vi "Vessel Operation.vi"() -> ()   [LabVIEW 2017, in "Saturation.lvclass"]
uses:
  Saturation.lvclass
  Type Defs/Tank.ctl
  Type Defs/Saturation State.ctl
  Process Settings/Process Settings.lvclass
  Process Settings/Type Defs/Item.ctl
  Type Defs/Valve State.ctl
  Process Settings/Type Defs/Units.ctl
panel:
  out "Elapsed Time":dbl(slide) scale=0.0..60.0
  in  "Stop":bool
  in  "Start":bool
  out "Temperature (bottom)":dbl
  out "Temperature (middle)":dbl
  out "Temperature (top)":dbl
  in  "Pressure Sensor Enabled":bool
  in  "Temperature (bottom) Enabled":bool
  in  "Temperature (middle) Enabled":bool
  in  "Temperature (top) Enabled":bool
  out "Tank pressure":T1 scale=0.0..100.0
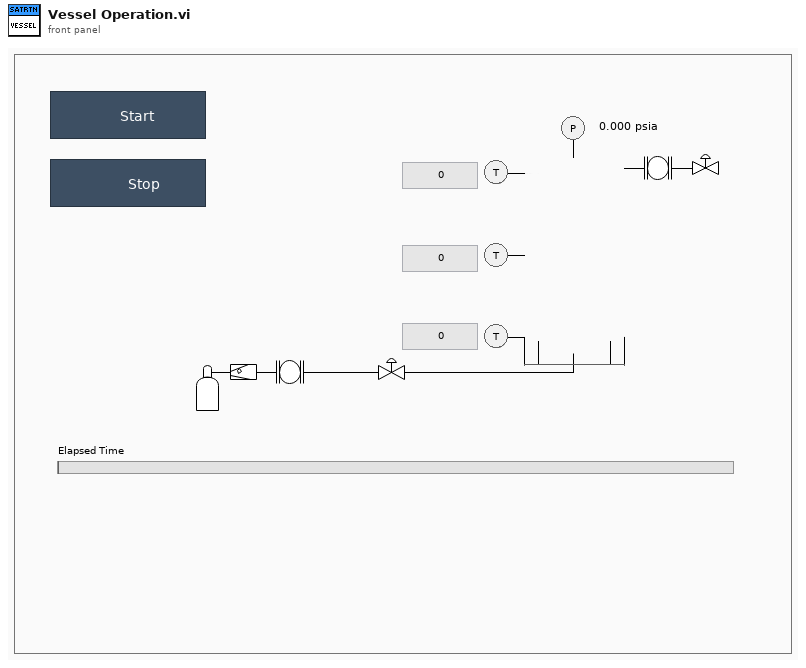
[diagram p1: front panel]
types:
  T1 = typedef "Saturation.lvclass/Tank.ctl" = dbl
  T2 = typedef "Saturation.lvclass/Saturation State.ctl" = enum16{"Init", "Update", "Go", "Control Valve", "Wait for Pressure", "Wait and Monitor", "Stop", "Idle", "Error", "Shutdown"}
  T3 = enum32{"Bad", "Idle", "Run top level", "Running"}
  T4 = typedef "Saturation.lvclass/Valve State.ctl" = enum16{"Fill", "Saturate", "Exhaust"}
  T5 = typedef "Process Settings.lvclass/Item.ctl" = enum16{"", "sheet temperature setpoint", "sheet heating time", "temp element setpoint", "chamber pressure setpoint", "saturation time", "chamber pressure valve setpoint"}
  T6 = typedef "Process Settings.lvclass/Units.ctl" = enum16{"°F", "°C", "Seconds", "Minutes", "PSIA", "V"}
  T7 = typedef "Saturation.lvclass/Saturation Temps.ctl" = cluster{"Tank Top Temp":dbl, "Tank Middle Temp":dbl, "Tank Bottom Temp":dbl}
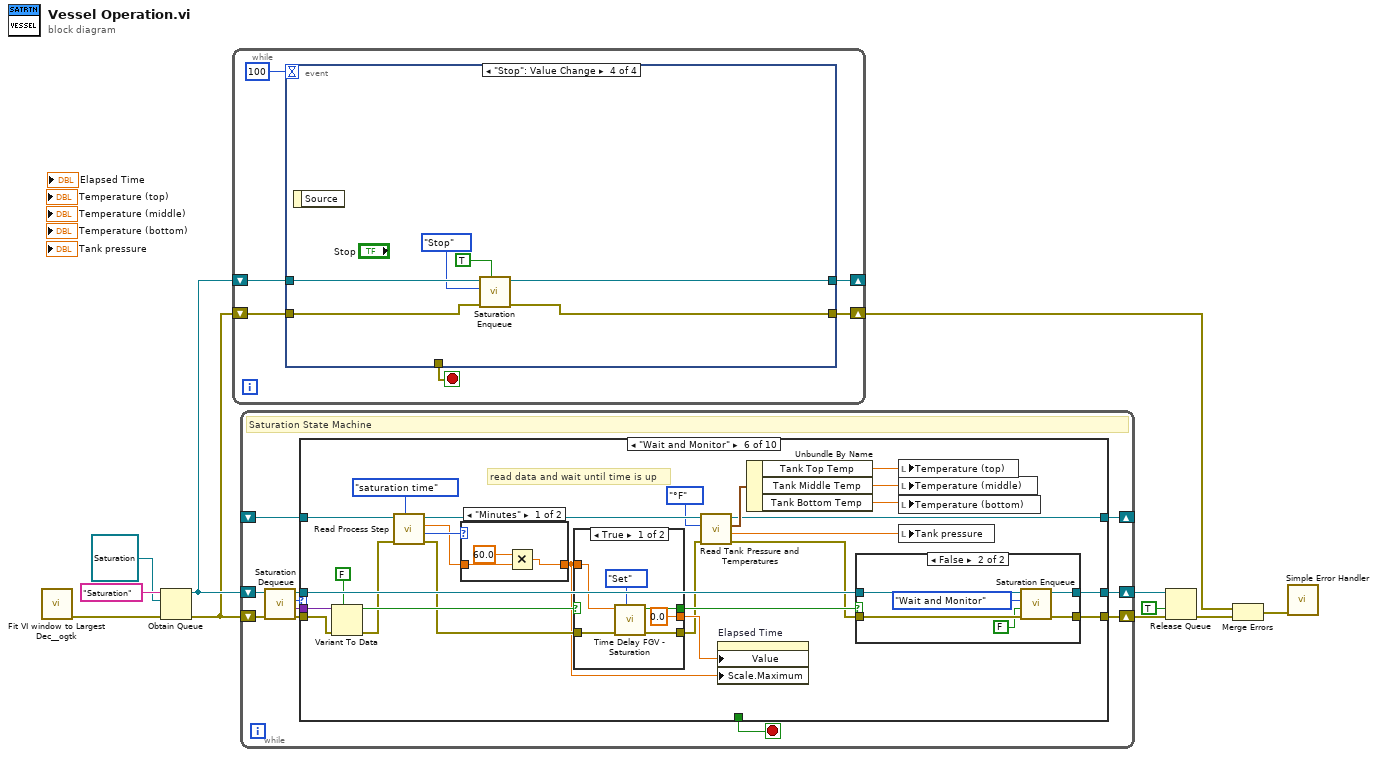
[diagram p0: block diagram]
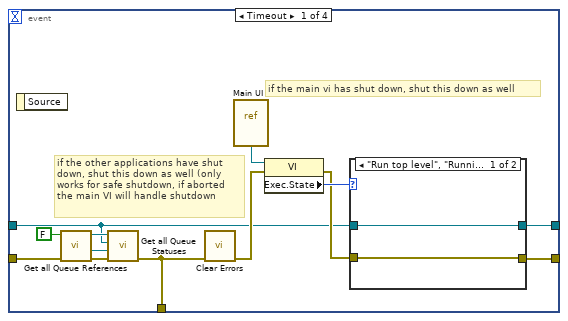
[diagram p2: hidden frame]
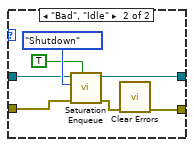
[diagram p3: hidden frame]
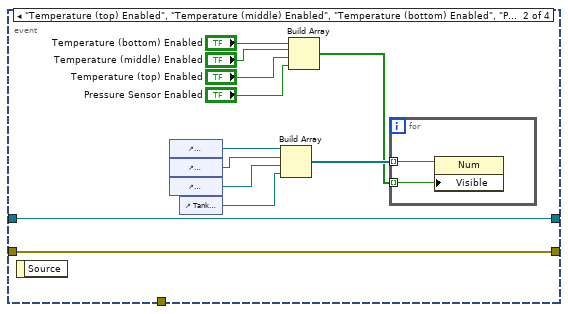
[diagram p4: hidden frame]
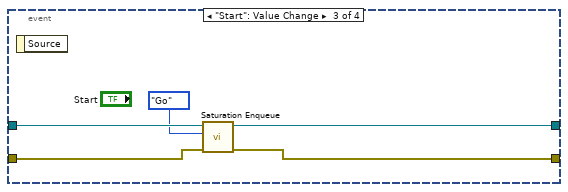
[diagram p5: hidden frame]
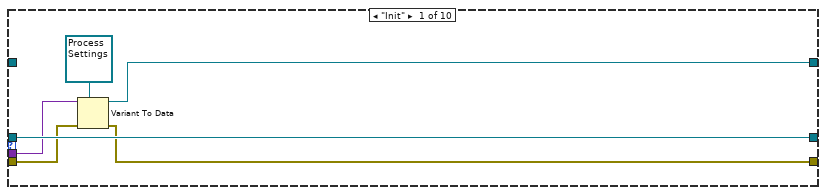
[diagram p6: hidden frame]
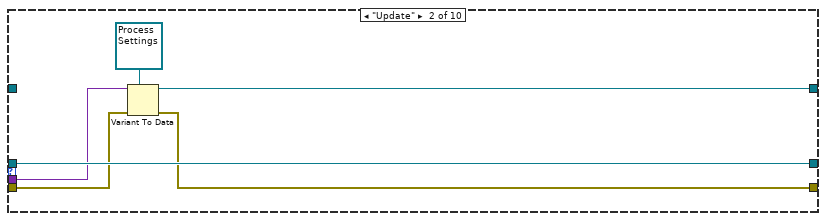
[diagram p7: hidden frame]
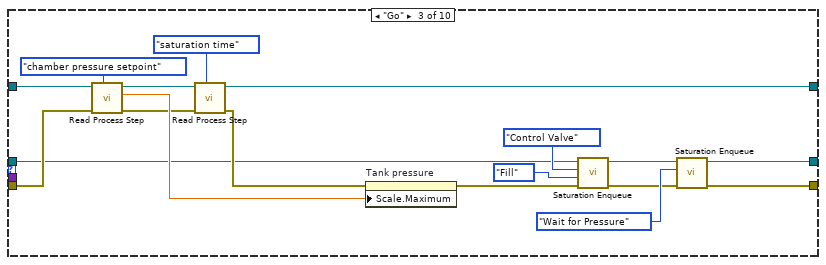
[diagram p8: hidden frame]
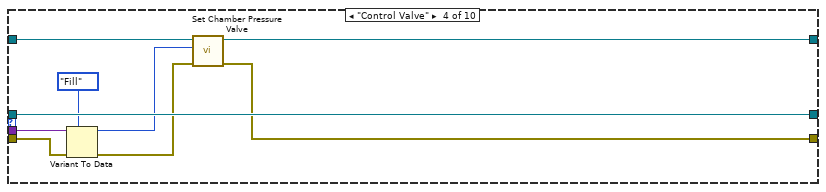
[diagram p9: hidden frame]
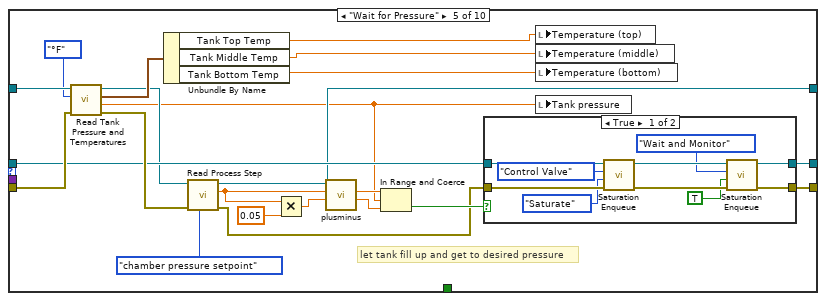
[diagram p10: hidden frame]
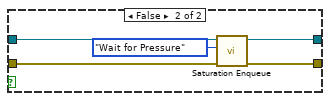
[diagram p11: hidden frame]
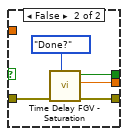
[diagram p13: hidden frame]
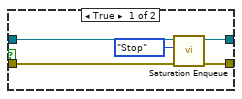
[diagram p14: hidden frame]
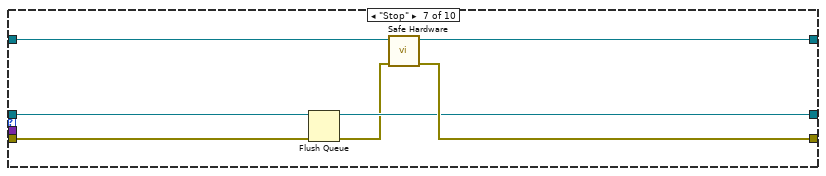
[diagram p15: hidden frame]
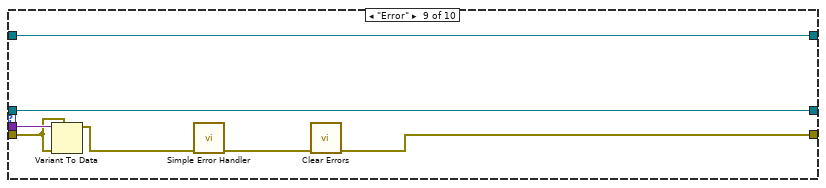
[diagram p17: hidden frame]
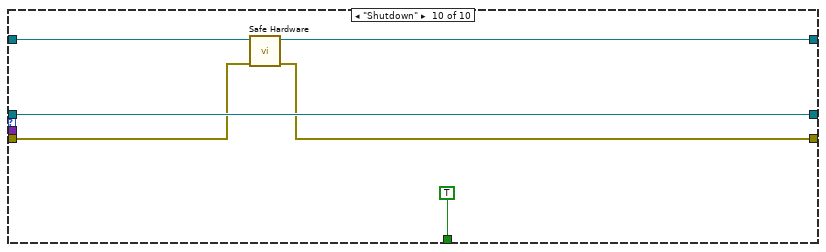
[diagram p18: hidden frame]
diagram:
  n1 = call <userlib>:"Fit VI window to Largest Dec__ogtk.vi"() -> ("error out"=w8:errorcluster)  [unwired: 6 in, 1 out]
  n2 = Obtain Queue(name (unnamed)="Saturation", element data type=refnum<class "Saturation.lvclass"> refnum ("Expansion.lvclass"), error in (no error)=w8) -> (queue out=w5:refnum<queue>, error out=w1:errorcluster)  [unwired: 2 in, 1 out]
  n3 = while {
    shift-right: [w14] -> w3
    shift-left: w1 -> [w16]
    shift-right: [w13] -> _
    shift-left: w5 -> [w17]
    stop <- w15 stop-if-true
    n4 = event shown="[3] \"Stop\": Value Change" {
      selector: _ -> [_ _ _ _]
      dyn-events: _ -> [_ _ _ _]
      timeout: 100 -> [_ _ _ _]
      tunnel: w17 -> [w19 w50 w58 w64]
      tunnel: w16 -> [w26 w51 w56 w62]
      tunnel: [w18 _ _ _] -> w15
      tunnel: [w20 w51 w55 w61] -> w14
      tunnel: [w21 w50 w57 w63] -> w13
      event Timeout {
        # "if the other applications have shut down, shut this down as well (only works for safe shutdown, if aborted the main VI will handle shutdown"
        # "if the main vi has shut down, shut this down as well"
        n5 = event-data() -> ()  [unwired: 1 in, 1 out]
        n6 = call "Get all Queue References.vi"("error in (no error)"=w26, "create if not found? (F)"=FALSE ("create if not found? (T)")) -> ("error out"=w29:errorcluster, "Recipes Queue"=w30:refnum<queue>, "Expansion Queue"=w27:refnum<queue>)  [unwired: 6 in, 1 out]
        n7 = call "Get all Queue Statuses.vi"("error in (no error)"=w29, "Recipes Queue"=w30, "Saturation Queue"=w19, "Expansion Queue"=w27) -> ("error out"=w18:errorcluster)  [unwired: 7 in]
        n8 = call <vilib>:"Clear Errors.vi"("error in (no error)"=w18) -> ("error out"=w23:errorcluster)  [unwired: 5 in, 1 out]
        n9 = vi-ref "Main UI.vi"() -> (w25:refnum<vi>)
        n10 = property class="VI"(reference=w25, error in=w23) -> (error out=w22:errorcluster, "Exec.State"=w24:T3)  [unwired: 1 out]
        n11 = case shown="\"Run top level\", \"Running\"" w24 {
          tunnel: w19 -> [w32 w35]
          tunnel: [w32 w39] -> w21
          tunnel: [w31 w33] -> w20
          tunnel: w22 -> [w31 w37]
          frame "Run top level", "Running" {
          }
          frame "Bad", "Idle" {
            n12 = call "Saturation Enqueue.vi"("Opposite End?"=TRUE, "error in (no error)"=w37, "State"=Saturation_State."Shutdown", "Queue in"=w35) -> ("error out"=w38:errorcluster, "Queue out"=w39:refnum<queue>)  [unwired: 6 in]
            n13 = call <vilib>:"Clear Errors.vi"("error in (no error)"=w38) -> ("error out"=w33:errorcluster)  [unwired: 5 in, 1 out]
          }
        }
      }
      event "Temperature (top) Enabled", "Temperature (middle) Enabled", "Temperature (bottom) Enabled", "Pressure Sensor Enabled": Value Change {
        n14 = event-data() -> ()  [unwired: 1 in, 1 out]
        n15 = control-ref of="Temperature (bottom)"() -> (w49:refnum<vi>)
        n16 = control-ref of="Temperature (middle)"() -> (w48:refnum<vi>)
        n17 = control-ref of="Temperature (top)"() -> (w47:refnum<vi>)
        n18 = control-ref of="Tank pressure"() -> (w46:refnum<vi>)
        n19 = Build Array(w49, w48, w47, w46) -> (w41:refnum<vi>[])
        n20 = Build Array("Temperature (bottom) Enabled", "Temperature (middle) Enabled", "Temperature (top) Enabled", "Pressure Sensor Enabled") -> (w40:bool[])
        n21 = for {
          tunnel: w41 -> [w53] mode=indexing
          tunnel: w40 -> [w52] mode=indexing
          n22 = property class="Num"(reference=w53, "Visible"=w52) -> ()  [unwired: 1 in, 2 out]
        }
      }
      event "Start": Value Change {
        n23 = event-data() -> ()  [unwired: 1 in, 1 out]
        n24 = call "Saturation Enqueue.vi"("error in (no error)"=w56, "State"=Saturation_State."Go", "Queue in"=w58) -> ("error out"=w55:errorcluster, "Queue out"=w57:refnum<queue>)  [unwired: 7 in]
      }
      event "Stop": Value Change {
        n25 = event-data() -> ()  [unwired: 1 in, 1 out]
        n26 = call "Saturation Enqueue.vi"("Opposite End?"=TRUE, "error in (no error)"=w62, "State"=Saturation_State."Stop", "Queue in"=w64) -> ("error out"=w61:errorcluster, "Queue out"=w63:refnum<queue>)  [unwired: 6 in]
      }
    }
  }
  n27 = while {
    shift-right: [w71] -> w10
    shift-left: w1 -> [w74]
    shift-right: [w69] -> w11
    shift-left: w5 -> [w75]
    shift-right: [w66] -> _
    shift-left: _ -> [w65]
    stop <- w70 stop-if-true
    # "Saturation State Machine"
    n28 = call "Saturation Dequeue.vi"("error in (no error)"=w74, "Queue in"=w75) -> ("error out"=w72:errorcluster, "Data"=w67:variant, "State"=w68:T2, "Queue out"=w73:refnum<queue>)  [unwired: 6 in]
    n29 = case shown="\"Wait and Monitor\"" w68 {
      tunnel: w73 -> [w81 w87 w95 w114 w120 w177 w210 w212 w220 w226]
      tunnel: w72 -> [w77 w82 w105 w111 w135 w173 w205 w213 w216 w222]
      tunnel: [w76 w84 w90 w107 w125 w175 w207 w213 w219 w221] -> w71
      tunnel: [_ _ _ _ _ _ _ _ _ TRUE] -> w70
      tunnel: [w81 w87 w92 w114 w126 w176 w206 w212 w220 w226] -> w69
      tunnel: w67 -> [w79 w85 _ w113 _ w174 _ _ w218 _]
      tunnel: [w78 w83 w98 w108 w117 w157 w208 w211 w215 w223] -> w66
      tunnel: w65 -> [_ _ w99 w109 w134 w168 w209 w211 w215 w224]
      frame "Init" {
        n30 = Variant To Data(error in=w77, type=refnum<class "Process Settings.lvclass"> refnum ("Process Settings.lvclass"), Variant=w79) -> (data=w78:refnum<class "Process Settings.lvclass">, error out=w76:errorcluster)
      }
      frame "Update" {
        n31 = Variant To Data(error in=w82, type=refnum<class "Process Settings.lvclass"> refnum ("Process Settings.lvclass"), Variant=w85) -> (data=w83:refnum<class "Process Settings.lvclass">, error out=w84:errorcluster)
      }
      frame "Go" {
        n32 = call "Read Process Step.vi"("Item"=Item."chamber pressure setpoint", "error in (no error)"=w105, "Process Settings in"=w99) -> ("error out"=w97:errorcluster, "Value"=w103:dbl, "Process Settings out"=w101:refnum<class "Process Settings.lvclass">)  [unwired: 5 in, 1 out]
        n33 = call "Read Process Step.vi"("Item"=Item."saturation time", "error in (no error)"=w97, "Process Settings in"=w101) -> ("error out"=w96:errorcluster, "Process Settings out"=w98:refnum<class "Process Settings.lvclass">)  [unwired: 5 in, 2 out]
        n34 = property on="Tank pressure" class="Slide (strict)"(error in=w96, "Scale.Maximum"=w103) -> (error out=w94:errorcluster)  [unwired: 1 in, 1 out]
        n35 = call "Saturation Enqueue.vi"("error in (no error)"=w94, "Data"=Valve_State."Fill" ("Open/Closed"), "State"=Saturation_State."Control Valve", "Queue in"=w95) -> ("error out"=w89:errorcluster, "Queue out"=w93:refnum<queue>)  [unwired: 6 in]
        n36 = call "Saturation Enqueue.vi"("error in (no error)"=w89, "State"=Saturation_State."Wait for Pressure", "Queue in"=w93) -> ("error out"=w90:errorcluster, "Queue out"=w92:refnum<queue>)  [unwired: 7 in]
      }
      frame "Control Valve" {
        n37 = Variant To Data(error in=w111, type=Valve_State."Fill" ("Open/Closed"), Variant=w113) -> (data=w110:T4, error out=w106:errorcluster)
        n38 = call "Set Chamber Pressure Valve.vi"("error in (no error)"=w106, "State"=w110, "Process Settings in"=w109) -> ("error out"=w107:errorcluster, "Process Settings out"=w108:refnum<class "Process Settings.lvclass">)  [unwired: 7 in]
      }
      frame "Wait for Pressure" {
        # "let tank fill up and get to desired pressure"
        n39 = call "Read Tank Pressure and Temperatures.vi"("error in (no error)"=w135, "Temp Units"=Units."°F", "Process Settings in"=w134) -> ("error out"=w121:errorcluster, "Tank Pressure"=w115:dbl, "Tank Temperature Cluster"=w136:T7, "Process Settings out"=w118:refnum<class "Process Settings.lvclass">)  [unwired: 5 in]
        n40 = Unbundle By Name(w136) -> ("Tank Top Temp"=w122:dbl, "Tank Middle Temp"=w123:dbl, "Tank Bottom Temp"=w124:dbl)
        n41 = call "Read Process Step.vi"("Item"=Item."chamber pressure setpoint", "error in (no error)"=w121, "Process Settings in"=w118) -> ("error out"=w119:errorcluster, "Value"=w130:dbl, "Process Settings out"=w117:refnum<class "Process Settings.lvclass">)  [unwired: 5 in, 1 out]
        n42 = Multiply(x=w130, y=0.05) -> (x*y=w131:dbl)
        n43 = call "plusminus.vi"("y"=w131, "x"=w130) -> ("x - y"=w128:dbl, "x + y"=w129:dbl)  [unwired: 4 in]
        n44 = In Range and Coerce(upper limit=w129, x=w115, lower limit=w128) -> (In Range?=w127:bool)  [unwired: 1 out]
        n45 = case shown="True" w127 {
          tunnel: w120 -> [w146 w151]
          tunnel: [w141 w150] -> w126
          tunnel: w119 -> [w145 w149]
          tunnel: [w140 w148] -> w125
          frame True {
            n46 = call "Saturation Enqueue.vi"("error in (no error)"=w145, "Data"=Valve_State."Saturate" ("Open/Closed"), "State"=Saturation_State."Control Valve", "Queue in"=w146) -> ("error out"=w139:errorcluster, "Queue out"=w142:refnum<queue>)  [unwired: 6 in]
            n47 = call "Saturation Enqueue.vi"("error in (no error)"=w139, "Data"=TRUE, "State"=Saturation_State."Wait and Monitor", "Queue in"=w142) -> ("error out"=w140:errorcluster, "Queue out"=w141:refnum<queue>)  [unwired: 6 in]
          }
          frame False {
            n48 = call "Saturation Enqueue.vi"("error in (no error)"=w149, "State"=Saturation_State."Wait for Pressure", "Queue in"=w151) -> ("error out"=w148:errorcluster, "Queue out"=w150:refnum<queue>)  [unwired: 7 in]
          }
        }
        n49 = local write "Temperature (top)"(w122) -> ()
        n50 = local write "Temperature (middle)"(w123) -> ()
        n51 = local write "Temperature (bottom)"(w124) -> ()
        n52 = local write "Tank pressure"(w115) -> ()
      }
      frame "Wait and Monitor" {
        # "read data and wait until time is up"
        n53 = Variant To Data(error in=w173, type=FALSE, Variant=w174) -> (data=w170:bool, error out=w167:errorcluster)
        n54 = call "Read Process Step.vi"("Item"=Item."saturation time", "error in (no error)"=w167, "Process Settings in"=w168) -> ("error out"=w166:errorcluster, "Units"=w160:T6, "Value"=w159:dbl, "Process Settings out"=w158:refnum<class "Process Settings.lvclass">)  [unwired: 5 in]
        n55 = case shown="\"Minutes\"" w160 {
          tunnel: w159 -> [w180 w181]
          tunnel: [w179 w181] -> w152
          frame "Minutes" {
            n56 = Multiply(x=60.0, y=w180) -> (x*y=w179:dbl)
          }
          frame "Seconds", Default {
          }
        }
        n57 = case shown="True" w170 {
          tunnel: w166 -> [w187 w192]
          tunnel: [w186 w191] -> w154
          tunnel: [0.0 ("Elapsed Time") w188] -> w155
          tunnel: [w184 w189] -> w171
          tunnel: w152 -> [w183 _]
          frame True {
            n58 = call "Time Delay FGV - Saturation.vi"("State"=enum16{"Set", "Done?"}."Set", "error in (no error)"=w187, "Time to wait (s)"=w183) -> ("error out"=w186:errorcluster, "Time's Up!"=w184:bool)  [unwired: 6 in, 1 out]
          }
          frame False {
            n59 = call "Time Delay FGV - Saturation.vi"("State"=enum16{"Set", "Done?"}."Done?", "error in (no error)"=w192) -> ("error out"=w191:errorcluster, "Elapsed Time"=w188:dbl, "Time's Up!"=w189:bool)  [unwired: 7 in]
          }
        }
        n60 = call "Read Tank Pressure and Temperatures.vi"("error in (no error)"=w154, "Temp Units"=Units."°F", "Process Settings in"=w158) -> ("error out"=w153:errorcluster, "Tank Pressure"=w164:dbl, "Tank Temperature Cluster"=w165:T7, "Process Settings out"=w157:refnum<class "Process Settings.lvclass">)  [unwired: 5 in]
        n61 = property on="Elapsed Time" class="Slide (strict)"("Value"=w155, "Scale.Maximum"=w152) -> ()  [unwired: 2 in, 2 out]
        n62 = Unbundle By Name(w165) -> ("Tank Top Temp"=w161:dbl, "Tank Middle Temp"=w162:dbl, "Tank Bottom Temp"=w163:dbl)
        n63 = case shown="False" w171 {
          tunnel: w177 -> [w197 w203]
          tunnel: [w196 w202] -> w176
          tunnel: w153 -> [w195 w201]
          tunnel: [w194 w200] -> w175
          frame True {
            n64 = call "Saturation Enqueue.vi"("error in (no error)"=w195, "State"=Saturation_State."Stop", "Queue in"=w197) -> ("error out"=w194:errorcluster, "Queue out"=w196:refnum<queue>)  [unwired: 7 in]
          }
          frame False {
            n65 = call "Saturation Enqueue.vi"("error in (no error)"=w201, "Data"=FALSE, "State"=Saturation_State."Wait and Monitor", "Queue in"=w203) -> ("error out"=w200:errorcluster, "Queue out"=w202:refnum<queue>)  [unwired: 6 in]
          }
        }
        n66 = local write "Temperature (top)"(w161) -> ()
        n67 = local write "Temperature (middle)"(w162) -> ()
        n68 = local write "Temperature (bottom)"(w163) -> ()
        n69 = local write "Tank pressure"(w164) -> ()
      }
      frame "Stop" {
        n70 = Flush Queue(queue=w210, error in (no error)=w205) -> (queue out=w206:refnum<queue>, error out=w204:errorcluster)  [unwired: 1 out]
        n71 = call "Safe Hardware.vi"("error in (no error)"=w204, "Process Settings in"=w209) -> ("error out"=w207:errorcluster, "Process Settings out"=w208:refnum<class "Process Settings.lvclass">)  [unwired: 8 in]
      }
      frame "Idle" {
      }
      frame "Error" {
        n72 = Variant To Data(error in=w216, type=w216, Variant=w218) -> (data=w217:errorcluster)  [unwired: 1 out]
        n73 = call <vilib>:"Simple Error Handler.vi"("error in (no error)"=w217) -> ("error out"=w214:errorcluster)  [unwired: 4 in, 4 out]
        n74 = call <vilib>:"Clear Errors.vi"("error in (no error)"=w214) -> ("error out"=w219:errorcluster)  [unwired: 5 in, 1 out]
      }
      frame "Shutdown" {
        n75 = call "Safe Hardware.vi"("error in (no error)"=w222, "Process Settings in"=w224) -> ("error out"=w221:errorcluster, "Process Settings out"=w223:refnum<class "Process Settings.lvclass">)  [unwired: 8 in]
      }
    }
  }
  n76 = Release Queue(queue=w11, force destroy? (F)=TRUE, error in (no error)=w10) -> (error out=w6:errorcluster)  [unwired: 2 out]
  n77 = Merge Errors(w3, w6) -> (w2:errorcluster)
  n78 = call <vilib>:"Simple Error Handler.vi"("error in (no error)"=w2) -> ()  [unwired: 4 in, 5 out]
